vi "Import IO Controls.vi"(8 "error in (no error)":errorcluster, 11 "Node Ptr":u64 format="%.0x") -> (0 "error out":errorcluster)   [LabVIEW 2024, in "Diagnostics Addon System Explorer.lvlib"]
uses:
  Diagnostics Addon System Explorer.lvlib
  Types/IO.Export.ctl
  Types/CmdResp.Export.ctl
  Addon Shared/Types/Signal.ctl
  Addon Shared/Types/Type.ctl
  <vilib>/Utility/error.llb/Trim Whitespace One-Sided.vi
  Addon Shared/Diagnostics Addon Shared.lvlib
  <vilib>/NI VeriStand/Custom Device Tools/Custom Device Utility Library/Custom Device Utility Library.lvlib
  <vilib>/NI VeriStand/Custom Device API/Custom Device API.lvlib
panel:
  in  "Tag":string
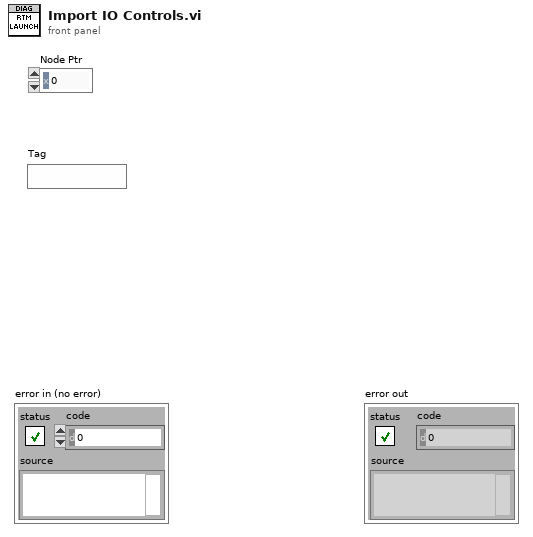
[diagram p1: front panel]
types:
  T1 = typedef "Diagnostics Addon System Explorer.lvlib/IO.Export.ctl" = cluster{"Name":string, "ID":u16, "Signals":T2}
  T2 = typedef "Diagnostics Addon System Explorer.lvlib/CmdResp.Export.ctl" = cluster{"Cmd":T3[], "Response":T3[]}
  T3 = typedef "Diagnostics Addon Shared.lvlib/Signal.ctl" = cluster{"Start Bit":u32, "Length":u32, "Scaling Factor":dbl, "Scaling Offset":dbl, "Minimum":dbl, "Maximum":dbl, "Data Type":u32, "Byte Order":u32, "Default Value":dbl, "Name":string, "Units":string}
  T4 = typedef "Diagnostics Addon Shared.lvlib/Type.ctl" = enum16{"DID", "CDID", "PID", "CPID", "Read Memory", "Write Memory", "IO Control", "Routine Start", "Routine Request", "Routine Stop", "User Defined", "DTC Control", "Clear DTCs", "Read DTCs", "Start DTCs", "DTC Change Count", "Tester Present", "Unlock ECU", "Reset ECU", "Diag Session Control", "Communication Control", "DPID Control", "Poll Control", "Diag Comm Port Control"}
  T5 = typedef "Custom Device API.lvlib/Custom Device Item Ref.ctl" = u64
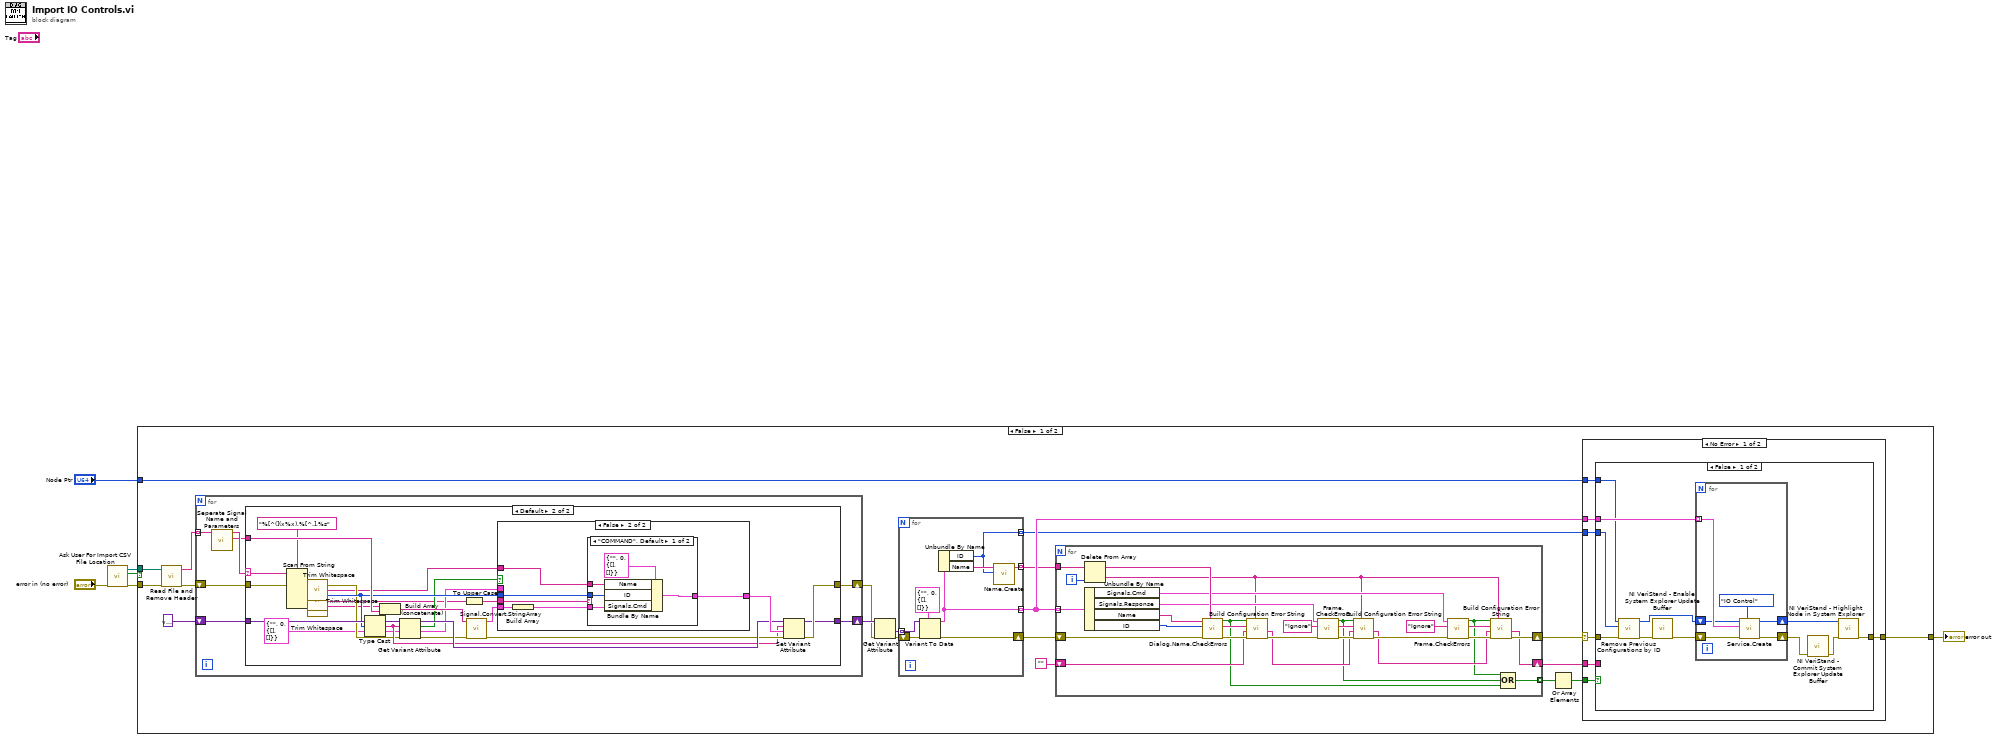
[diagram p0: block diagram]
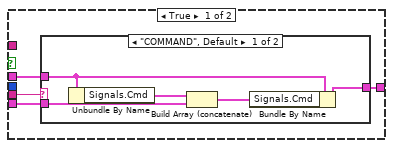
[diagram p3: hidden frame]
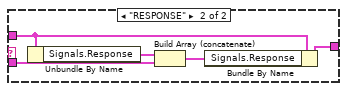
[diagram p4: hidden frame]
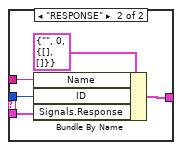
[diagram p5: hidden frame]
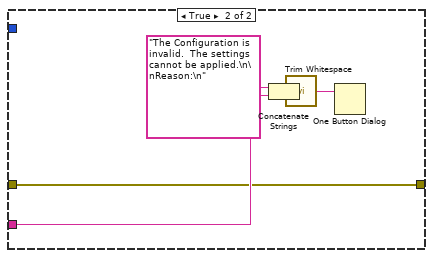
[diagram p6: hidden frame]
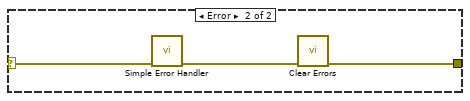
[diagram p7: hidden frame]
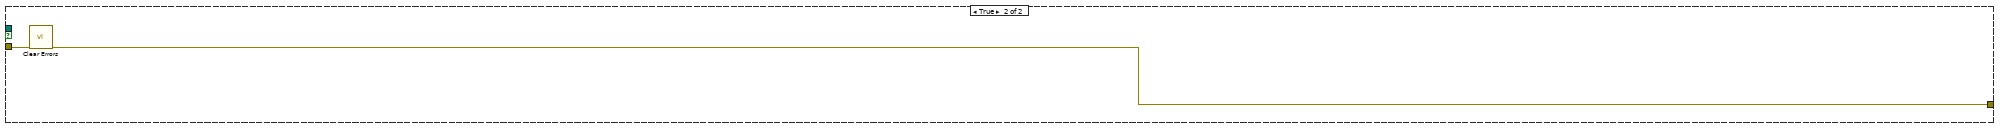
[diagram p8: hidden frame]
diagram:
  n1 = call "Ask User For Import CSV File Location.vi"("error in (no error)"="error in (no error)") -> ("error out"=w2:errorcluster, "cancelled"=w3:bool, "selected path"=w1:path)  [unwired: 8 in]
  n2 = case shown="False" w3 {
    tunnel: w2 -> [w26 w162]
    tunnel: w1 -> [w25 _]
    tunnel: "Node Ptr" -> [w11 _]
    tunnel: [w13 w161] -> w5
    frame False {
      n3 = call "Read File and Remove Header.vi"("error in (no error)"=w26, "selected path"=w25) -> ("error out"=w24:errorcluster, "Array"=w8:string[])  [unwired: 8 in]
      n4 = for {
        tunnel: w8 -> [w33] mode=indexing
        shift-right: [w30] -> w21
        shift-left: w24 -> [w31]
        shift-right: [w29] -> w22
        shift-left: variant -> [w32]
        n5 = call "Seperate Signal Name and Parameters.vi"("String"=w33) -> ("Signal Parameters"=w27:string[], "Signal Name"=w28:string)  [unwired: 9 in]
        n6 = case shown="Default" w28 {
          selector: w28 -> [_ w44]
          tunnel: w27 -> [_ w61]
          tunnel: w32 -> [w35 w57]
          tunnel: w31 -> [w34 w56]
          tunnel: [w34 w51] -> w30
          tunnel: [w35 w50] -> w29
          frame "" {
          }
          frame Default {
            n7 = Scan From String(format string="%[^(](x%x).%[^.].%s", input string=w44, error in=w56) -> (error out=w48:errorcluster, output 1=w59:string, output 2=w55:u32, output 3=w41:string, output 4=w42:string)  [unwired: 5 in, 2 out]
            n8 = call <vilib>:"Trim Whitespace.vi"("string"=w59) -> ("trimmed string"=w38:string)  [unwired: 1 in]
            n9 = call <vilib>:"Trim Whitespace.vi"("string"=w41) -> ("trimmed string"=w37:string)  [unwired: 1 in]
            n10 = call <vilib>:"Trim Whitespace.vi"("string"=w42) -> ("trimmed string"=w36:string)  [unwired: 1 in]
            n11 = Type Cast(x=w55) -> (*(type *) &x=w49:string)  [unwired: 1 in]
            n12 = Build Array (concatenate)(w36, w61) -> (w58:string[])
            n13 = Get Variant Attribute(Variant=w57, name=w49, default value (empty Variant)=T1 {"Name"="", "ID"=0, "Signals"={"Cmd"=[], "Response"=[]}} ("IO Control"), error in=w48) -> (duplicate Variant=w53:variant, found=w46:bool, value=w45:T1, error out=w47:errorcluster)
            n14 = To Upper Case(1:w37) -> (0:w40:string)
            n15 = call "Signal.Convert.StringArray.vi"("error in (no error)"=w47, "Signal Parameters"=w58) -> ("error out"=w52:errorcluster, "Signal Parameters"=w60:T3)  [unwired: 8 in]
            n16 = case shown="False" w46 {
              tunnel: w60 -> [w64 w81]
              tunnel: w38 -> [_ w80]
              tunnel: w55 -> [_ w78]
              tunnel: [w63 w77] -> w54
              tunnel: w45 -> [w65 _]
              tunnel: w40 -> [w62 w76]
              frame True {
                n17 = case shown="\"COMMAND\", Default" w62 {
                  tunnel: w65 -> [w70 w75]
                  tunnel: w64 -> [w68 w73]
                  tunnel: [w66 w71] -> w63
                  frame "COMMAND", Default {
                    n18 = Unbundle By Name(w70) -> ("Signals.Cmd"=w69:T3[])
                    n19 = Build Array (concatenate)(w69, w68) -> (w67:T3[])
                    n20 = Bundle By Name(cluster=w70, "Signals.Cmd"=w67) -> (w66:T1)
                  }
                  frame "RESPONSE" {
                    n21 = Unbundle By Name(w75) -> ("Signals.Response"=w74:T3[])
                    n22 = Build Array (concatenate)(w74, w73) -> (w72:T3[])
                    n23 = Bundle By Name(cluster=w75, "Signals.Response"=w72) -> (w71:T1)
                  }
                }
              }
              frame False {
                n24 = Build Array(w81) -> (w79:T3[])
                n25 = case shown="\"COMMAND\", Default" w76 {
                  tunnel: w80 -> [w86 w91]
                  tunnel: w79 -> [w85 w90]
                  tunnel: w78 -> [w84 w89]
                  tunnel: [w83 w88] -> w77
                  frame "COMMAND", Default {
                    n26 = Bundle By Name(cluster=T1 {"Name"="", "ID"=0, "Signals"={"Cmd"=[], "Response"=[]}} ("IO Control"), "Name"=w86, "ID"=w84, "Signals.Cmd"=w85) -> (w83:T1)
                  }
                  frame "RESPONSE" {
                    n27 = Bundle By Name(cluster=T1 {"Name"="", "ID"=0, "Signals"={"Cmd"=[], "Response"=[]}} ("IO Control"), "Name"=w91, "ID"=w89, "Signals.Response"=w90) -> (w88:T1)
                  }
                }
              }
            }
            n28 = Set Variant Attribute(Variant=w53, name=w49, value=w54, error in=w52) -> (Variant out=w50:variant, error out=w51:errorcluster)  [unwired: 1 out]
          }
        }
      }
      n29 = Get Variant Attribute(Variant=w22, error in=w21) -> (values=w20:variant[], error out=w19:errorcluster)  [unwired: 2 in, 2 out]
      n30 = for {
        tunnel: w20 -> [w99] mode=indexing
        shift-right: [w97] -> w12
        shift-left: w19 -> [w98]
        tunnel: [w96] -> w14 mode=indexing
        tunnel: [w92] -> w10 mode=indexing
        tunnel: [w94] -> w7 mode=indexing
        n31 = Variant To Data(error in=w98, type=T1 {"Name"="", "ID"=0, "Signals"={"Cmd"=[], "Response"=[]}} ("IO Control"), Variant=w99) -> (data=w96:T1, error out=w97:errorcluster)
        n32 = Unbundle By Name(w96) -> ("ID"=w92:u16, "Name"=w95:string)
        n33 = call "Name.Create.vi"("PID Number"=w92, "PID Name"=w95) -> ("VS Name"=w94:string)  [unwired: 9 in]
      }
      n34 = for {
        tunnel: w14 -> [w128] mode=indexing
        shift-right: [w127] -> w9
        shift-left: w12 -> [w121]
        shift-right: [w106] -> w15
        shift-left: "" -> [w109]
        tunnel: [w104] -> w17 mode=indexing
        tunnel: w7 -> [w126]
        i -> [w125]
        n35 = Delete From Array(array=w126, index=w125) -> (deleted portion=w102:string, array with subset deleted=w124:string[])  [unwired: 1 in]
        n36 = Unbundle By Name(w128) -> ("Signals.Cmd"=w118:T3[], "Signals.Response"=w120:T3[], "Name"=w123:string, "ID"=w122:u16)
        n37 = call "Dialog.Name.CheckErrors.vi"("Existing Frames"=w124, "error in (no error)"=w121, "ID"=w122, "Name"=w123) -> ("error out"=w116:errorcluster, "Error"=w115:string, "Error?"=w100:bool)  [unwired: 5 in]
        n38 = call "Build Configuration Error String.vi"("Name"=w102, "error in (no error)"=w116, "String in"=w109, "Error"=w115, "Error?"=w100) -> ("error out"=w114:errorcluster, "String out"=w108:string)  [unwired: 5 in]
        n39 = call "Frame.CheckErrors.vi"("error in (no error)"=w114, "Name"="Ignore", "Signals"=w120) -> ("error out"=w113:errorcluster, "Error Type"=w112:string, "Error?"=w105:bool)  [unwired: 6 in]
        n40 = call "Build Configuration Error String.vi"("Name"=w102, "error in (no error)"=w113, "String in"=w108, "Error"=w112, "Error?"=w105) -> ("error out"=w111:errorcluster, "String out"=w107:string)  [unwired: 5 in]
        n41 = call "Frame.CheckErrors.vi"("error in (no error)"=w111, "Name"="Ignore", "Signals"=w118) -> ("error out"=w119:errorcluster, "Error Type"=w110:string, "Error?"=w101:bool)  [unwired: 6 in]
        n42 = call "Build Configuration Error String.vi"("Name"=w102, "error in (no error)"=w119, "String in"=w107, "Error"=w110, "Error?"=w101) -> ("error out"=w127:errorcluster, "String out"=w106:string)  [unwired: 5 in]
        n43 = Compound Arithmetic op=OR(w101, w105, w100) -> (w104:bool)
      }
      n44 = Or Array Elements(Boolean array=w17) -> (logical OR=w16:bool)
      n45 = case shown="No Error" w9 {
        selector: w9 -> [w131 w160]
        tunnel: w16 -> [w135 _]
        tunnel: w15 -> [w134 _]
        tunnel: w14 -> [w133 _]
        tunnel: [w132 w158] -> w13
        tunnel: w11 -> [w130 _]
        tunnel: w10 -> [w129 _]
        frame No Error {
          n46 = case shown="False" w135 {
            tunnel: w134 -> [_ w155]
            tunnel: w131 -> [w139 w154]
            tunnel: w133 -> [w142 _]
            tunnel: [w141 w154] -> w132
            tunnel: w130 -> [w138 _]
            tunnel: w129 -> [w140 _]
            frame False {
              n47 = call "Remove Previous Configurations by ID.vi"("error in (no error)"=w139, "Imported IDs"=w140, "Node In"=w138) -> ("error out"=w137:errorcluster, "Node Out"=w136:T5)  [unwired: 7 in]
              n48 = call <vilib>:"NI VeriStand - Enable System Explorer Update Buffer.vi"("error in (no error)"=w137) -> ("error out"=w145:errorcluster)  [unwired: 10 in]
              n49 = for {
                shift-right: [w149] -> w144
                shift-left: w145 -> [w148]
                shift-right: [w150] -> w146
                shift-left: w136 -> [w151]
                tunnel: w142 -> [w152] mode=indexing
                n50 = call "Service.Create.vi"("Type"=Type."IO Control", "error in (no error)"=w148, "Variant"=w152, "Section Ptr"=w151) -> ("error out"=w149:errorcluster, "Parent Ref out"=w150:T5)  [unwired: 6 in]
              }
              n51 = call <vilib>:"NI VeriStand - Commit System Explorer Update Buffer.vi"("error in (no error)"=w144) -> ("error out"=w143:errorcluster)  [unwired: 10 in]
              n52 = call <vilib>:"NI VeriStand - Highlight Node in System Explorer.vi"("error in (no error)"=w143, "Item Ref in"=w146) -> ("error out"=w141:errorcluster)  [unwired: 8 in, 1 out]
            }
            frame True {
              n53 = Concatenate Strings("The Configuration is invalid.  The settings cannot be applied.\n\nReason:\n" ("message"), w155) -> (w157:string)
              n54 = call <vilib>:"Trim Whitespace.vi"("string"=w157) -> ("trimmed string"=w153:string)  [unwired: 1 in]
              n55 = One Button Dialog(message=w153) -> ()  [unwired: 1 in, 1 out]
            }
          }
        }
        frame Error {
          n56 = call <vilib>:"Simple Error Handler.vi"("error in (no error)"=w160) -> ("error out"=w159:errorcluster)  [unwired: 4 in, 4 out]
          n57 = call <vilib>:"Clear Errors.vi"("error in (no error)"=w159) -> ("error out"=w158:errorcluster)  [unwired: 5 in, 1 out]
        }
      }
    }
    frame True {
      n58 = call <vilib>:"Clear Errors.vi"("error in (no error)"=w162) -> ("error out"=w161:errorcluster)  [unwired: 5 in, 1 out]
    }
  }
  "error out" <- w5
